vi "robo_waitx.vi"(2 "tick":i32, 4 "错误输入（无错误）":errorcluster, 5 "tmo":i32, 6 "dst":i32, 7 "page":i32, 8 "ax":i32, 9 "VISA资源名称":refnum<visa-resource-name>) -> (0 "错误输出":errorcluster, 1 "f":i32, 3 "VISA资源名称输出":refnum<visa-resource-name>)   [LabVIEW 2017]
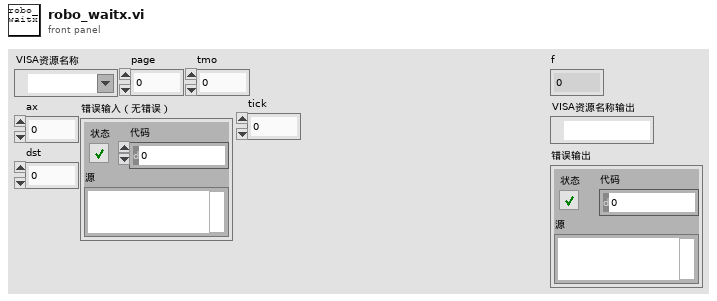
[diagram p1: front panel]
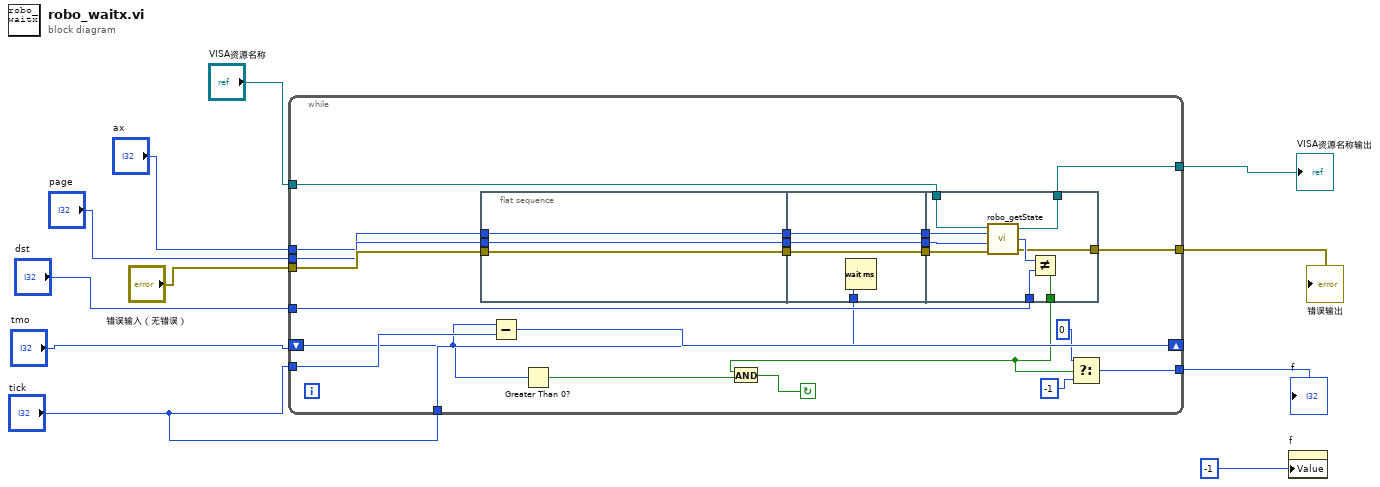
[diagram p0: block diagram]
diagram:
  n1 = while {
    tunnel: "tick" -> [w34]
    shift-right: [w33] -> _
    shift-left: "tmo" -> [w22]
    tunnel: "错误输入（无错误）" -> [w32]
    tunnel: "page" -> [w31]
    tunnel: "ax" -> [w30]
    tunnel: "VISA资源名称" -> [w29]
    tunnel: [w28] -> w2
    tunnel: "dst" -> [w27]
    tunnel: "tick" -> [w23]
    tunnel: [w13] -> w4
    tunnel: [w12] -> w1
    stop <- w20 continue-if-true
    n2 = flat-sequence {
      tunnel: w30 -> [w35]
      tunnel: w31 -> [w36]
      tunnel: w32 -> [w37]
      tunnel: [w37] -> w19
      tunnel: [w36] -> w18
      tunnel: [w35] -> w17
      tunnel: [w41] -> w26
      tunnel: [w40] -> w25
      tunnel: [w39] -> w24
      tunnel: w23 -> [w38]
      tunnel: w19 -> [w41]
      tunnel: w18 -> [w40]
      tunnel: w17 -> [w39]
      tunnel: w29 -> [w47]
      tunnel: [w46] -> w28
      tunnel: w27 -> [w44]
      tunnel: w26 -> [w50]
      tunnel: w25 -> [w49]
      tunnel: w24 -> [w48]
      tunnel: [w43] -> w16
      tunnel: [w42] -> w12
      frame #0 {
      }
      frame #1 {
        n3 = Wait (ms)(milliseconds to wait=w38) -> ()  [unwired: 1 out]
      }
      frame #2 {
        n4 = call "robo_getState.vi"("错误输入（无错误）"=w50, "输入 2"=w49, "输入 1"=w48, "VISA资源名称"=w47) -> ("错误输出"=w42:errorcluster, "数字"=w45:i32, "VISA资源名称输出"=w46:refnum<visa-resource-name>)
        n5 = Not Equal?(x=w45, y=w44) -> (x != y?=w43:bool)
      }
    }
    n6 = Subtract(x=w22, y=w34) -> (x-y=w33:i32)
    n7 = Greater Than 0?(x=w22) -> (x > 0?=w21:bool)
    n8 = And(x=w16, y=w21) -> (x .and. y?=w20:bool)
    n9 = Select(t=0, s=w16, f=-1) -> (s? t:f=w13:i32)
  }
  "f" <- w4
  "VISA资源名称输出" <- w2
  "错误输出" <- w1
  n10 = property on="f" class="DigNum (严格)"("Value"=-1 ("f")) -> ()  [unwired: 2 in, 2 out]
